vi "Init.vi"(6 "Template Path":path, 8 "Project:Active Project":refnum<vi>, 9 "Application Instance":refnum<vi>, 10 "Template Name":string) -> (3 "Script out":refnum<class "Script.lvclass">)   [LabVIEW 2021, in "_Template.lvlib" / "Script.lvlib" / "Script.lvclass"]
uses:
  Script.lvclass
  Script.lvclass/Script.ctl
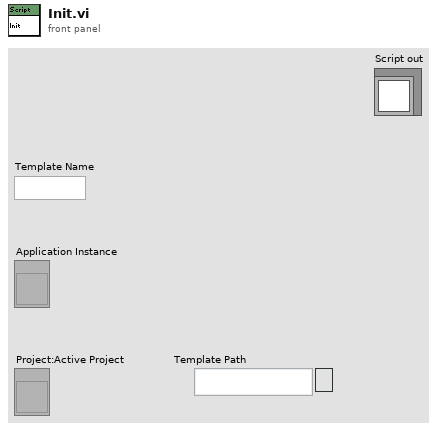
[diagram p1: front panel]
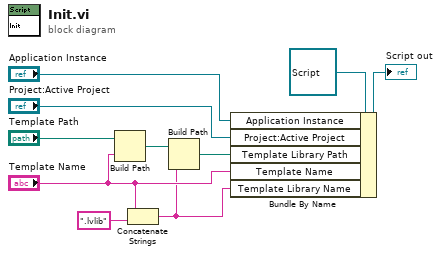
[diagram p0: block diagram]
diagram:
  n1 = Build Path(base path="Template Path", name or relative path="Template Name") -> (appended path=w7:path)
  n2 = Concatenate Strings("Template Name", ".lvlib" ("string")) -> (w2:string)
  n3 = Build Path(base path=w7, name or relative path=w2) -> (appended path=w5:path)
  n4 = Bundle By Name(cluster=refnum<class "Script.lvclass"> refnum ("_Create From Template.lvlib:Script Strategy.lvlib:First Library Script Strategy.lvclass"), "Application Instance"="Application Instance", "Project:Active Project"="Project:Active Project", "Template Library Path"=w5, "Template Name"="Template Name", "Template Library Name"=w2) -> (→"Script out":refnum<class "Script.lvclass">)
